vi "MicroZed Version.vi"(3 "Version Numeric":u16) -> (1 "Version String":string)   [LabVIEW 2014]
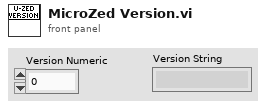
[diagram p1: front panel]
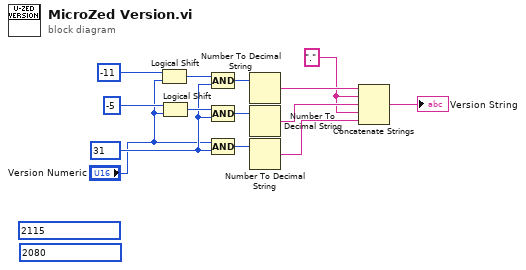
[diagram p0: block diagram]
diagram:
  (unwired) u16 2080
  w4 = "."
  w8 = u16 31 ("value")
  (unwired) u16 2115
  n1 = Logical Shift(y=i16 -11, x="Version Numeric") -> (x << y=w9:u16)
  n2 = Logical Shift(y=i16 -5, x="Version Numeric") -> (x << y=w11:u16)
  n3 = Compound Arithmetic op=AND(w9, w8) -> (w7:u16)
  n4 = Compound Arithmetic op=AND(w11, w8) -> (w13:u16)
  n5 = Compound Arithmetic op=AND("Version Numeric", w8) -> (w14:u16)
  n6 = Number To Decimal String(number=w7) -> (decimal integer string=w6:string)  [unwired: 1 in]
  n7 = Number To Decimal String(number=w13) -> (decimal integer string=w5:string)  [unwired: 1 in]
  n8 = Number To Decimal String(number=w14) -> (decimal integer string=w3:string)  [unwired: 1 in]
  n9 = Concatenate Strings(w6, w4, w5, w4, w3) -> (→"Version String":string)
